vi "FormatQueryString.vi"(0 "reference in":refnum<class "TelegramBOT.lvclass">, 2 "QueryStringIn":string, 4 "QueryStringItems":T1[](array[typedef]), 5 "error in (no error)":errorcluster) -> (14 "reference out":refnum<class "TelegramBOT.lvclass">, 16 "QueryStringOut":string, 19 "error out":errorcluster)   [LabVIEW 2014, in "TelegramBOT.lvclass"]
uses:
  TelegramBOT.lvclass
  QueryStringElem.ctl
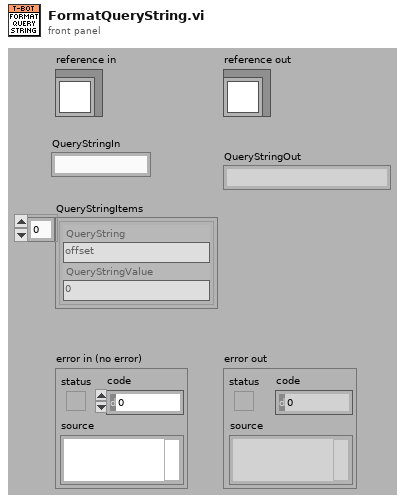
[diagram p1: front panel]
types:
  T1 = typedef "TelegramBOT.lvclass/QueryStringElem.ctl" = cluster{"QueryString":string, "QueryStringValue":string}
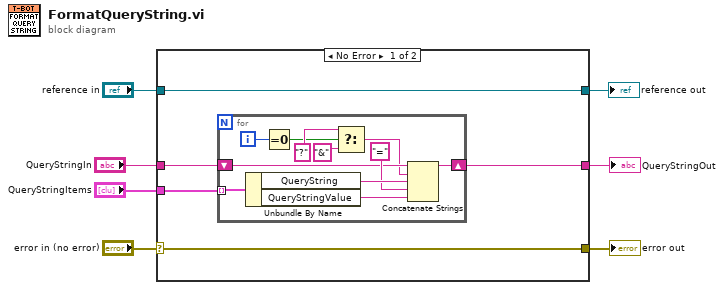
[diagram p0: block diagram]
diagram:
  n1 = case shown="No Error" "error in (no error)" {
    selector: "error in (no error)" -> [w11 w25]
    tunnel: [w11 w25] -> w6
    tunnel: [w12 w24] -> w4
    tunnel: "reference in" -> [w12 w24]
    tunnel: [w10 _] -> w3
    tunnel: "QueryStringIn" -> [w9 _]
    tunnel: "QueryStringItems" -> [w8 _]
    frame No Error {
      n2 = for {
        tunnel: w8 -> [w22] mode=indexing
        shift-right: [w23] -> w10
        shift-left: w9 -> [w14]
        i -> [w16]
        n3 = Unbundle By Name(w22) -> ("QueryString"=w19:string, "QueryStringValue"=w17:string)
        n4 = Equal To 0?(x=w16) -> (x = 0?=w15:bool)
        n5 = Select(t="?", s=w15, f="&") -> (s? t:f=w13:string)
        n6 = Concatenate Strings(w14, w13, w19, "=", w17) -> (w23:string)
      }
    }
    frame Error {
    }
  }
  "error out" <- w6
  "reference out" <- w4
  "QueryStringOut" <- w3
